vi "sub_verifyPuzzle.vi"(8 "error in (no error)":errorcluster, 11 "row (in)":string[](array[string])) -> (0 "error out":errorcluster, 2 "solved ?":bool)   [LabVIEW 2018]
panel:
  out "invalid row ?":bool
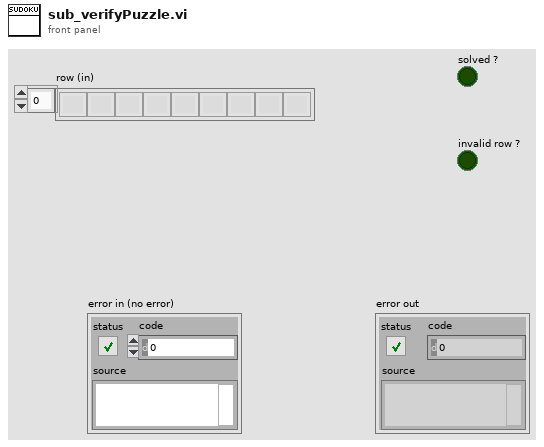
[diagram p1: front panel]
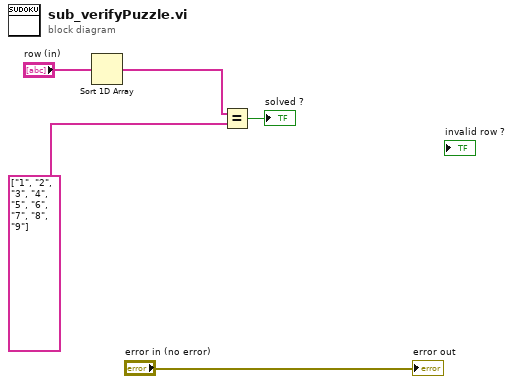
[diagram p0: block diagram]
diagram:
  n1 = Sort 1D Array(array="row (in)") -> (sorted array=w4:string[])
  n2 = Equal?(x=w4, y=string[] ["1", "2", "3", "4", "5", "6", "7", "8", "9"]) -> (x = y?=→"solved ?":bool)
  "error out" <- "error in (no error)"
